vi "Compile and Export Settings.vi"(8 "error in (no error)":errorcluster, 11 "Device Item Ref in":T1 format="%.0x") -> (0 "error out":errorcluster)   [LabVIEW 2015, in "Protection and Counter Addon System Explorer.lvlib"]
uses:
  Protection and Counter Addon System Explorer.lvlib
  <vilib>/NI Veristand/Custom Device API/Custom Device Item Ref.ctl
  Shared/Types/Exported.OnCompile.ctl
  Shared/Types/XNET Settings.ctl
  SubModules/Frame Protection Support/Source/Shared/Types/Exported Frame Settings.ctl
  SubModules/Frame Protection Support/Source/Shared/Types/Exported Frame Type.ctl
  SubModules/Frame Protection Support/Source/Shared/Types/Exported Protection Settings.ctl
  SubModules/Frame Protection Support/Source/Shared/Types/Protection Type.ctl
  SubModules/Frame Protection Support/Source/Shared/Types/XNET Signal Configuration.ctl
  SubModules/Frame Protection Support/Source/Shared/Types/Exported Counter Settings.ctl
  SubModules/Frame Protection Support/Source/Shared/Types/Exported Event Trigger Type.ctl
  Shared/Types/986x.ctl
  SubModules/Frame Protection Support/Source/Shared/Types/Incoming Signal Info.ctl
  SubModules/Frame Protection Support/Source/Shared/Types/Exported Signal Settings.ctl
  SubModules/Frame Protection Support/Source/System Explorer/Types/Export Frame GUIDs List.ctl
  <vilib>/NI Veristand/Custom Device Tools/Custom Device Utility Library/Search Direction.ctl
  SubModules/Frame Protection Support/Source/System Explorer/Types/Export Frames List and Type.ctl
  SubModules/Frame Protection Support/Source/System Explorer/Types/Exported Frame Settings.ctl
  Shared/SubVIs/GUID Lookup.vi
  <vilib>/NI Veristand/Custom Device API/NI VeriStand - Get Item Property.vi
  <vilib>/NI Veristand/Custom Device API/Get Item Property (Boolean).vi
  <vilib>/NI Veristand/Custom Device API/Get Item Property (String).vi
  FileDependency.Get.Target Path.vi
  <vilib>/NI Veristand/Custom Device Tools/Custom Device Utility Library/NI VeriStand - Search for All Items by GUID.vi
  <vilib>/NI Veristand/Custom Device Tools/Custom Device Utility Library/NI VeriStand - Search for Item by GUID.vi
  <vilib>/NI Veristand/Custom Device API/Set Item Property (Variant).vi
  <vilib>/NI VeriStand/Custom Device Tools/Custom Device Utility Library/Custom Device Utility Library.lvlib
  Shared/Protection and Counter Addon Shared.lvlib
  <vilib>/NI VeriStand/Custom Device API/Custom Device API.lvlib
  SubModules/Frame Protection Support/Source/Shared/Protection and Counter Support Shared.lvlib
  <vilib>/NI/NIVS Inline Async API/_Data Access System Explorer/Data Access System Explorer.lvlib
  SubModules/Frame Protection Support/Source/System Explorer/Protection and Counter Support System Explorer.lvlib
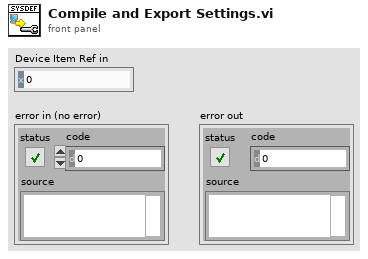
[diagram p1: front panel]
types:
  T1 = typedef "Custom Device API.lvlib/Custom Device Item Ref.ctl" = u64
  T2 = cluster{"Name":string, "Type":enum16{"Output/Write", "Input/Read", "Input/ReadWrite"}, "VS Refs":T1[]}
  T3 = typedef "Protection and Counter Support System Explorer.lvlib/Export Frames List and Type.ctl" = cluster{"Type":T4, "Frame Refs":T1[], "Frame Settings":T5[]}
  T4 = typedef "Protection and Counter Support Shared.lvlib/Exported Frame Type.ctl" = enum16{"Periodic", "Event", "Periodic/Event"}
  T5 = typedef "Protection and Counter Support System Explorer.lvlib/Exported Frame Settings.ctl" = cluster{"ID":u32, "Disable Transmission":bool, "Disable Transmission Ref":T1, "Transmit Trigger":T6, "Transmit Trigger Ref":T1}
  T6 = typedef "Protection and Counter Support Shared.lvlib/Exported Event Trigger Type.ctl" = enum16{"Channel value change", "Trigger channel (not zero)", "Channel value change or trigger channel (not zero)", "Trigger channel (any value change)", "Channel value change or trigger channel (any value change)"}
  T7 = typedef "Custom Device Utility Library.lvlib/Search Direction.ctl" = enum16{"Down", "Up"}
  T8 = typedef "Protection and Counter Support System Explorer.lvlib/Export Frame GUIDs List.ctl" = cluster{"Signal Page GUID":string, "Rolling Counter Value GUID":string, "Protection Value GUID":string}
  T9 = typedef "Protection and Counter Addon Shared.lvlib/Exported.OnCompile.ctl" = cluster{"XNET Settings":T10, "Frames":T11[], "986x Support":T16, "Incoming Frames":T11[], "Incoming Signal Info":T17}
  T10 = typedef "Protection and Counter Addon Shared.lvlib/XNET Settings.ctl" = cluster{"Database":refnum<k21>, "Cluster":refnum<k21>, "Port":string, "Baud rate [Bd]":u64, "Termination":u32, "CAN I/O Mode":u32, "FD Baud rate [Bd]":u64, "Priority":i32, "Use Legacy":bool}
  T11 = typedef "Protection and Counter Support Shared.lvlib/Exported Frame Settings.ctl" = cluster{"Type":T4, "Frame ID":u32, "Payload Length":u32, "Signal XNET Paths":string[], "Frame.PrevData":dbl[], "VS Offset":i32, "VS Length":i32, "Generation Period":u32, "Has Protection?":bool, "Protection Configurations":T12[], "Has Counter":bool, "Counter Configurations":T15[], "Has Disable?":bool, "Disable VS Index":i32, "Transmit Trigger":T6, "Trigger VS Index":i32}
  T12 = typedef "Protection and Counter Support Shared.lvlib/Exported Protection Settings.ctl" = cluster{"Protection Frame Index":i32, "Protection Type":T13, "Data Indeces":i32[], "Initialized Data Array":dbl[], "Protection Signal XNET Paths":string[], "CRC Channels":T14[], "Protection VS Update Index":i32}
  T13 = typedef "Protection and Counter Support Shared.lvlib/Protection Type.ctl" = enum16{"Arb ID + Bytes Checksum with Inversion", "Arb ID + Bytes CRC with Inversion", "Reversed Raw Signal Checksum with Inversion"}
  T14 = typedef "Protection and Counter Support Shared.lvlib/XNET Signal Configuration.ctl" = cluster{"Start Bit":i32, "Name":string, "Number of bits":i32, "Scale":dbl, "Offset":dbl, "Data Type":u32}
  T15 = typedef "Protection and Counter Support Shared.lvlib/Exported Counter Settings.ctl" = cluster{"Counter Frame Index":i32, "Max Count":dbl, "Counter VS Index":i32}
  T16 = typedef "Protection and Counter Addon Shared.lvlib/986x.ctl" = cluster{"Enable":bool, "RIO Device":string, "Bitfile":path}
  T17 = typedef "Protection and Counter Support Shared.lvlib/Incoming Signal Info.ctl" = cluster{"Signal Settings Out":T18[], "Signal.PrevData":dbl[], "Signal Names":string[]}
  T18 = typedef "Protection and Counter Support Shared.lvlib/Exported Signal Settings.ctl" = cluster{"Is Protection":bool, "Is Counter":bool, "Signal Name":string, "Counter Configuration":T15, "Protection Configuration":T12, "Valid_Sig_Ref_Index":i32}
  T19 = typedef "Protection and Counter Addon System Explorer.lvlib/Frame Settings.ctl" = cluster{"ID":u32, "Disable Transmission":bool, "Disable Transmission Ref":T1, "Transmit Trigger":T20, "Transmit Trigger Ref":T1}
  T20 = typedef "Protection and Counter Addon System Explorer.lvlib/Event Trigger Type.ctl" = enum16{"Channel value change", "Trigger channel (not zero)", "Channel value change or trigger channel (not zero)", "Trigger channel (any value change)", "Channel value change or trigger channel (any value change)"}
  T21 = cluster{"Name":string, "Type":enum16{"Output/Write", "Input/Read", "Input/ReadWrite"}, "VS Refs":T1[]}[]
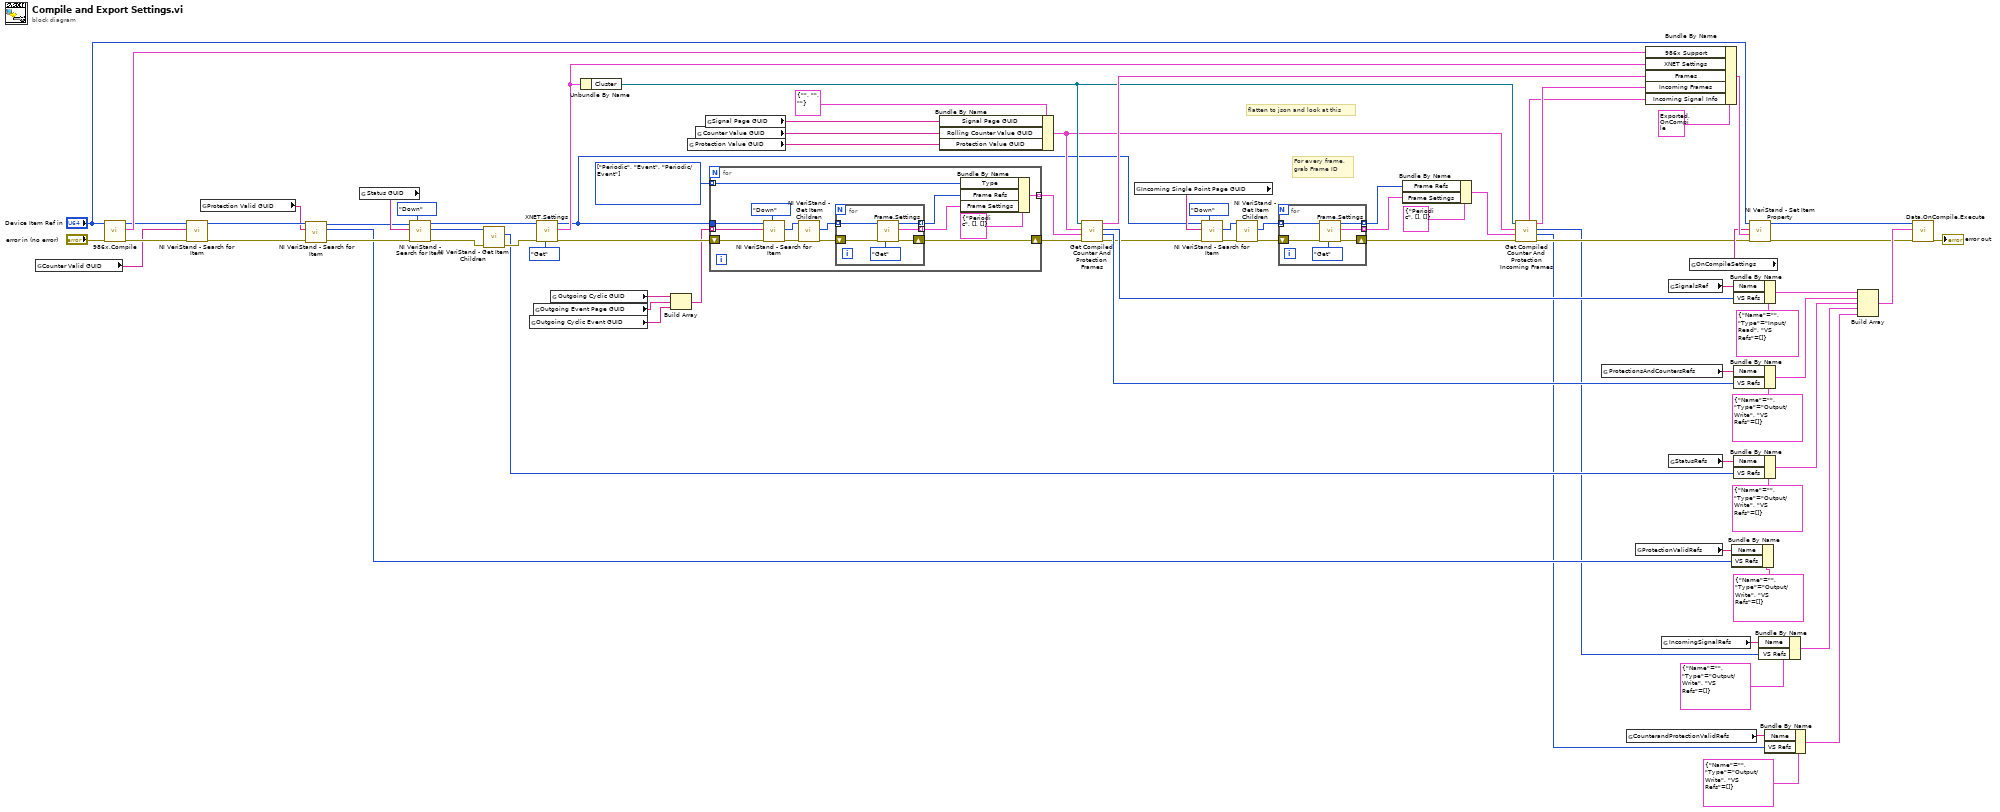
[diagram p0: block diagram]
diagram:
  w49 = T4[] [enum."Periodic", enum."Event", enum."Periodic/Event"] items=["Periodic", "Event", "Periodic/Event"]
  # "For every frame,\ngrab Frame ID"
  # "flatten to json and look at this"
  n1 = global read "GUID Lookup.vi" "Counter Valid GUID"() -> (w35:string)
  n2 = call "986x.Compile.vi"("error in (no error)"="error in (no error)", "Item Ref in"="Device Item Ref in") -> ("error out"=w37:errorcluster, "986x Support"=w46:T16, "Item Ref out"=w36:T1)  [unwired: 7 in]
  n3 = call-poly <vilib>:"NI VeriStand - Search for Item.vi"("error in"=w37, "Item GUID"=w35, "Section Ref in"=w36) -> ("error out"=w30:errorcluster, "Section Ref out"=w34:T1)  [unwired: 5 in, 2 out]
  n4 = global read "GUID Lookup.vi" "Protection Valid GUID"() -> (w33:string)
  n5 = call-poly <vilib>:"NI VeriStand - Search for Item.vi"("error in"=w30, "Item GUID"=w33, "Section Ref in"=w34) -> ("error out"=w31:errorcluster, "Item Refs"=w26:T1[], "Section Ref out"=w32:T1)  [unwired: 5 in, 1 out]
  n6 = global read "GUID Lookup.vi" "Status GUID"() -> (w62:string)
  n7 = call-poly <vilib>:"NI VeriStand - Search for Item.vi"("Direction (Down)"=Search_Direction."Down", "error in"=w31, "Item GUID"=w62, "Section Ref in"=w32) -> ("error out"=w59:errorcluster, "Item Ref"=w60:T1, "Section Ref out"=w61:T1)  [unwired: 4 in, 1 out]
  n8 = call <vilib>:"NI VeriStand - Get Item Children.vi"("error in (no error)"=w59, "Item Ref in"=w60) -> ("error out"=w58:errorcluster, "Child Refs"=w57:T1[])  [unwired: 6 in, 2 out]
  n9 = global read "GUID Lookup.vi" "Outgoing Cyclic Event GUID"() -> (w40:string)
  n10 = global read "GUID Lookup.vi" "Outgoing Event Page GUID"() -> (w41:string)
  n11 = call "XNET.Settings.vi"("Action"=enum8{"Get", "Set"}."Get", "error in (no error)"=w58, "Parent Ref in"=w61) -> ("error out"=w39:errorcluster, "XNET Settings"=w78:T10, "Item Ref out"=w10:T1)  [unwired: 6 in]
  n12 = global read "GUID Lookup.vi" "Outgoing Cyclic GUID"() -> (w42:string)
  n13 = Unbundle By Name(w78) -> ("Cluster"=w12:refnum<k21>)
  n14 = Build Array(w42, w41, w40) -> (w38:string[])
  n15 = global read "GUID Lookup.vi" "Protection Value GUID"() -> (w52:string)
  n16 = global read "GUID Lookup.vi" "Counter Value GUID"() -> (w53:string)
  n17 = global read "GUID Lookup.vi" "Signal Page GUID"() -> (w54:string)
  n18 = for {
    shift-right: [w81] -> w50
    shift-left: w39 -> [w91]
    tunnel: w49 -> [w94] mode=indexing
    tunnel: [w93] -> w48 mode=indexing
    tunnel: w10 -> [w90]
    tunnel: w38 -> [w89] mode=indexing
    n19 = call-poly <vilib>:"NI VeriStand - Search for Item.vi"("Direction (Down)"=Search_Direction."Down", "error in"=w91, "Item GUID"=w89, "Section Ref in"=w90) -> ("error out"=w87:errorcluster, "Item Ref"=w88:T1)  [unwired: 4 in, 2 out]
    n20 = call <vilib>:"NI VeriStand - Get Item Children.vi"("error in (no error)"=w87, "Item Ref in"=w88) -> ("error out"=w85:errorcluster, "Child Refs"=w84:T1[])  [unwired: 6 in, 2 out]
    n21 = for {
      tunnel: w84 -> [w98] mode=indexing
      shift-right: [w97] -> w81
      shift-left: w85 -> [w99]
      tunnel: [w96] -> w83 mode=indexing
      tunnel: [w95] -> w82 mode=indexing
      n22 = call "Frame.Settings.vi"("Action"=enum8{"Get", "Set"}."Get", "error in (no error)"=w99, "Item Ref in"=w98) -> ("error out"=w97:errorcluster, "Frame.Settings"=w95:T19, "Item Ref out"=w96:T1)  [unwired: 6 in]
    }
    n23 = Bundle By Name(cluster=T3 {"Type"=enum."Periodic", "Frame Refs"=[], "Frame Settings"=[]} ("Export Frames List and Type"), "Type"=w94, "Frame Refs"=w83, "Frame Settings"=w82) -> (w93:T3)
  }
  n24 = Bundle By Name(cluster=T8 {"Signal Page GUID"="", "Rolling Counter Value GUID"="", "Protection Value GUID"=""}, "Signal Page GUID"=w54, "Rolling Counter Value GUID"=w53, "Protection Value GUID"=w52) -> (w11:T8)
  n25 = call "Get Compiled Counter And Protection Frames.vi"("error in (no error)"=w50, "Frames per type"=w48, "GUIDs"=w11, "XNET Cluster"=w12) -> ("error out"=w14:errorcluster, "Counters and Protection Refs"=w72:T1[], "Signals Refs"=w45:T1[], "Frames"=w44:T11[])  [unwired: 4 in]
  n26 = global read "GUID Lookup.vi" "Incoming Single Point Page GUID"() -> (w22:string)
  n27 = call-poly <vilib>:"NI VeriStand - Search for Item.vi"("Direction (Down)"=Search_Direction."Down", "error in"=w14, "Item GUID"=w22, "Section Ref in"=w10) -> ("error out"=w25:errorcluster, "Item Ref"=w24:T1)  [unwired: 4 in, 2 out]
  n28 = call <vilib>:"NI VeriStand - Get Item Children.vi"("error in (no error)"=w25, "Item Ref in"=w24) -> ("error out"=w17:errorcluster, "Child Refs"=w18:T1[])  [unwired: 6 in, 2 out]
  n29 = for {
    tunnel: w18 -> [w104] mode=indexing
    shift-right: [w103] -> w16
    shift-left: w17 -> [w105]
    tunnel: [w102] -> w20 mode=indexing
    tunnel: [w101] -> w19 mode=indexing
    n30 = call "Frame.Settings.vi"("Action"=enum8{"Get", "Set"}."Get", "error in (no error)"=w105, "Item Ref in"=w104) -> ("error out"=w103:errorcluster, "Frame.Settings"=w101:T19, "Item Ref out"=w102:T1)  [unwired: 6 in]
  }
  n31 = Bundle By Name(cluster=T3 {"Type"=enum."Periodic", "Frame Refs"=[], "Frame Settings"=[]} ("Export Frames List and Type"), "Frame Refs"=w20, "Frame Settings"=w19) -> (w15:T3)
  n32 = call "Get Compiled Counter And Protection Incoming Frames.vi"("error in (no error)"=w16, "Frames"=w15, "GUIDs"=w11, "XNET Cluster"=w12) -> ("error out"=w13:errorcluster, "Incoming Counters and Protection Valid Refs"=w3:T1[], "Incoming Signals Refs"=w8:T1[], "Incoming Frames"=w4:T11[], "Incoming Signal Info"=w1:T17)  [unwired: 3 in]
  n33 = global read "GUID Lookup.vi" "ProtectionsAndCountersRefs"() -> (w68:string)
  n34 = global read "GUID Lookup.vi" "CounterandProtectionValidRefs"() -> (w27:string)
  n35 = global read "GUID Lookup.vi" "ProtectionValidRefs"() -> (w28:string)
  n36 = Bundle By Name(cluster=T9 {"XNET Settings"={"Database"="", "Cluster"="", "Port"="", "Baud rate [Bd]"=500000, "Termination"=1, "CAN I/O Mode"=0, "FD Baud rate [Bd]"=500000, "Priority"=100, "Use Legacy"=FALSE}, "Frames"=[], "986x Support"={"Enable"=FALSE, "RIO Device"="", "Bitfile"=path ""}, "Incoming Frames"=[], "Incoming Signal Info"={"Signal Settings Out"=[], "Signal.PrevData"=[], "Signal Names"=[]}}, "986x Support"=w46, "XNET Settings"=w78, "Frames"=w44, "Incoming Frames"=w4, "Incoming Signal Info"=w1) -> (w77:T9)
  n37 = global read "GUID Lookup.vi" "IncomingSignalRefs"() -> (w9:string)
  n38 = global read "GUID Lookup.vi" "SignalsRef"() -> (w69:string)
  n39 = global read "GUID Lookup.vi" "StatusRefs"() -> (w64:string)
  n40 = global read "GUID Lookup.vi" "OnCompileSettings"() -> (w67:string)
  n41 = Bundle By Name(cluster=T2 {"Name"="", "Type"=enum."Output/Write", "VS Refs"=[]} ("Group"), "Name"=w28, "VS Refs"=w26) -> ()  [unwired: 1 out]
  n42 = Bundle By Name(cluster=T2 {"Name"="", "Type"=enum."Input/Read", "VS Refs"=[]} ("Group"), "Name"=w69, "VS Refs"=w45) -> (w75:T2)
  n43 = Bundle By Name(cluster=T2 {"Name"="", "Type"=enum."Output/Write", "VS Refs"=[]} ("Group"), "Name"=w68, "VS Refs"=w72) -> (w66:T2)
  n44 = Bundle By Name(cluster=T2 {"Name"="", "Type"=enum."Output/Write", "VS Refs"=[]} ("Group"), "Name"=w64, "VS Refs"=w57) -> (w47:T2)
  n45 = call-poly <vilib>:"NI VeriStand - Set Item Property.vi"("error in (no error)"=w13, "Value"=w77, "Property Name"=w67, "Item Ref in"="Device Item Ref in") -> ("error out"=w71:errorcluster, "Item Ref out"=w70:T1)  [unwired: 5 in, 1 out]
  n46 = Bundle By Name(cluster=T2 {"Name"="", "Type"=enum."Output/Write", "VS Refs"=[]} ("Group"), "Name"=w9, "VS Refs"=w8) -> (w5:T2)
  n47 = Bundle By Name(cluster=T2 {"Name"="", "Type"=enum."Output/Write", "VS Refs"=[]} ("Group"), "Name"=w27, "VS Refs"=w3) -> (w2:T2)
  n48 = Build Array(w75, w66, w47, w5, w2) -> (w74:T21)
  n49 = call <vilib>:"Data.OnCompile.Execute.vi"("error in"=w71, "VS Ref Groups"=w74, "Custom Device Ref"=w70) -> ("error out"=→"error out":errorcluster)  [unwired: 7 in, 1 out]
